vi "str2signal.vi"(3 "filter":bool=TRUE caption="Filter", 4 "srt in":string caption="cadena de entrada") -> (0 "sp":i32 caption="speed", 1 "v":cluster{"vx":dbl, "vy":dbl, "vy":dbl} caption="velocidad angular", 2 "a":cluster{"ax":dbl, "ay":dbl, "az":dbl} caption="aceleracion")   [LabVIEW 2019]
uses:
  <vilib>/ptbypt/NI_PtbyPt.lvlib
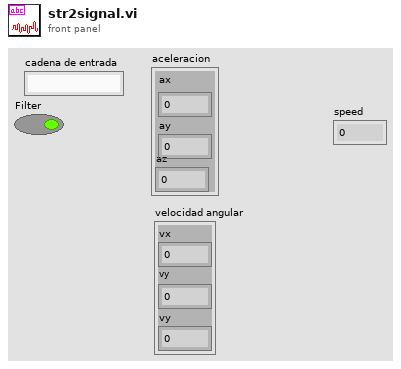
[diagram p1: front panel]
types:
  T1 = cluster{"Filtered x":dbl, "Filtered x":dbl, "Filtered x":dbl}
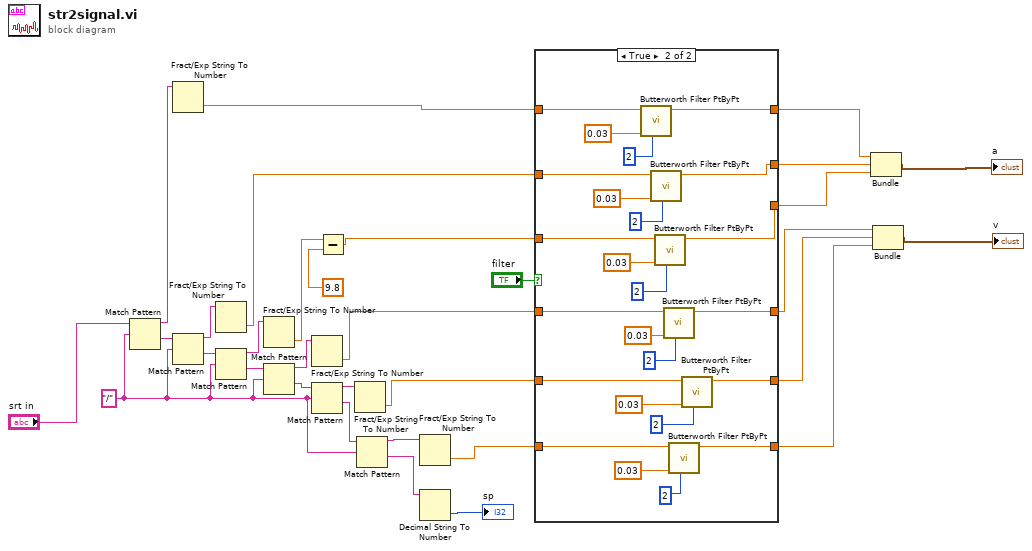
[diagram p0: block diagram]
diagram:
  w5 = "/" ("regular expression")
  n1 = Match Pattern(string="srt in", regular expression=w5) -> (before substring=w20:string, after substring=w19:string)  [unwired: 1 in, 2 out]
  n2 = Fract/Exp String To Number(string=w20) -> (number=w18:dbl)  [unwired: 3 in, 1 out]
  n3 = Match Pattern(string=w19, regular expression=w5) -> (before substring=w21:string, after substring=w22:string)  [unwired: 1 in, 2 out]
  n4 = Fract/Exp String To Number(string=w21) -> (number=w17:dbl)  [unwired: 3 in, 1 out]
  n5 = Match Pattern(string=w22, regular expression=w5) -> (before substring=w23:string, after substring=w24:string)  [unwired: 1 in, 2 out]
  n6 = Fract/Exp String To Number(string=w23) -> (number=w7:dbl)  [unwired: 3 in, 1 out]
  n7 = Match Pattern(string=w24, regular expression=w5) -> (before substring=w26:string, after substring=w25:string)  [unwired: 1 in, 2 out]
  n8 = Fract/Exp String To Number(string=w26) -> (number=w16:dbl)  [unwired: 3 in, 1 out]
  n9 = Match Pattern(string=w25, regular expression=w5) -> (before substring=w27:string, after substring=w6:string)  [unwired: 1 in, 2 out]
  n10 = Subtract(x=w7, y=9.8) -> (x-y=w8:dbl)
  n11 = Fract/Exp String To Number(string=w27) -> (number=w15:dbl)  [unwired: 3 in, 1 out]
  n12 = Match Pattern(string=w6, regular expression=w5) -> (before substring=w4:string, after substring=w3:string)  [unwired: 1 in, 2 out]
  n13 = Fract/Exp String To Number(string=w4) -> (number=w14:dbl)  [unwired: 3 in, 1 out]
  n14 = Decimal String To Number(string=w3) -> (number=→"sp":i32)  [unwired: 2 in, 1 out]
  n15 = case shown="True" "filter" {
    tunnel: [w33 w62] -> w32
    tunnel: w18 -> [w38 w49]
    tunnel: w17 -> [w37 w48]
    tunnel: w16 -> [w35 w47]
    tunnel: w15 -> [w34 w46]
    tunnel: w14 -> [w33 w45]
    tunnel: [w38 w44] -> w13
    tunnel: [w37 w43] -> w12
    tunnel: [w35 w42] -> w11
    tunnel: [w34 w41] -> w10
    tunnel: [w36 w40] -> w9
    tunnel: w8 -> [w36 w39]
    frame False {
    }
    frame True {
      n16 = call <vilib>:"Butterworth Filter PtByPt.vi"("order"=2, "low cutoff freq: fl"=0.03, "x"=w49) -> ("Filtered x"=w44:dbl)  [unwired: 6 in, 1 out]
      n17 = call <vilib>:"Butterworth Filter PtByPt.vi"("order"=2, "low cutoff freq: fl"=0.03, "x"=w48) -> ("Filtered x"=w43:dbl)  [unwired: 6 in, 1 out]
      n18 = call <vilib>:"Butterworth Filter PtByPt.vi"("order"=2, "low cutoff freq: fl"=0.03, "x"=w39) -> ("Filtered x"=w40:dbl)  [unwired: 6 in, 1 out]
      n19 = call <vilib>:"Butterworth Filter PtByPt.vi"("order"=2, "low cutoff freq: fl"=0.03, "x"=w47) -> ("Filtered x"=w42:dbl)  [unwired: 6 in, 1 out]
      n20 = call <vilib>:"Butterworth Filter PtByPt.vi"("order"=2, "low cutoff freq: fl"=0.03, "x"=w45) -> ("Filtered x"=w62:dbl)  [unwired: 6 in, 1 out]
      n21 = call <vilib>:"Butterworth Filter PtByPt.vi"("order"=2, "low cutoff freq: fl"=0.03, "x"=w46) -> ("Filtered x"=w41:dbl)  [unwired: 6 in, 1 out]
    }
  }
  n22 = Bundle("Filtered x"=w13, "Filtered x"=w12, "Filtered x"=w9) -> (→"a":T1)  [unwired: 1 in]
  n23 = Bundle("Filtered x"=w11, "Filtered x"=w10, "Filtered x"=w32) -> (→"v":T1)  [unwired: 1 in]
